vi "Dual to Double.vi"(1 "Dual":refnum<class "Dual.lvclass">) -> (0 "Double":dbl)   [LabVIEW 2020, in "Automatic Differentiation.lvlib" / "Dual.lvclass"]
uses:
  Dual.lvclass
  Dual.lvclass/Dual.ctl
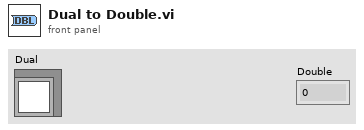
[diagram p1: front panel]
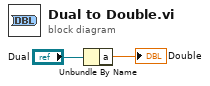
[diagram p0: block diagram]
diagram:
  n1 = Unbundle By Name("Dual") -> ("a"=→"Double":dbl)
